vi "testSHA384.vi"(8 "error in (no error)":errorcluster, 11 "TestCase in":refnum<class "TestHashing.lvclass">) -> (0 "error out":errorcluster, 3 "TestCase out":refnum<class "TestHashing.lvclass">)   [LabVIEW 2021, in "TestHashing.lvclass"]
uses:
  TestHashing.lvclass
  TestHashing.lvclass/TestHashing.ctl
  <vilib>/addons/_JKI Toolkits/VI Tester/TestCase.llb/TestCase.lvclass
  <vilib>/Wiresmith Technology/VITAC (VI Tester Advanced Comparisons)/VITAC.lvlib
  C:/Program Files (x86)/National Instruments/LabVIEW 2021/vi.lib/addons/_JKI Toolkits/VI Tester/TestCase.llb/TestCase.lvclass
  Hashing/dotNET Crypto Hashing.lvlib
  Utility/dotNET Crypto Utility.lvlib
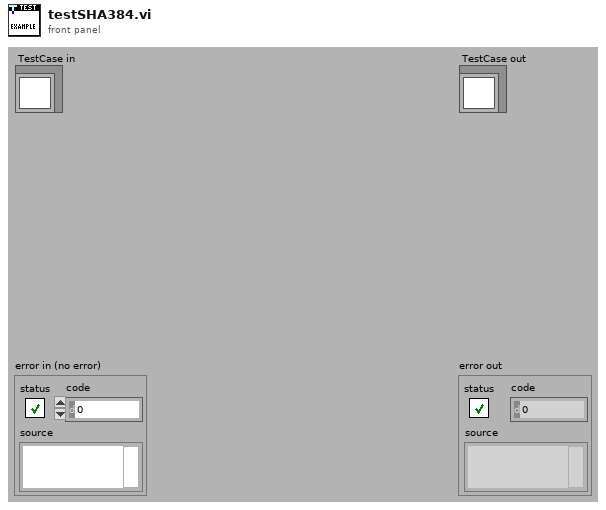
[diagram p1: front panel]
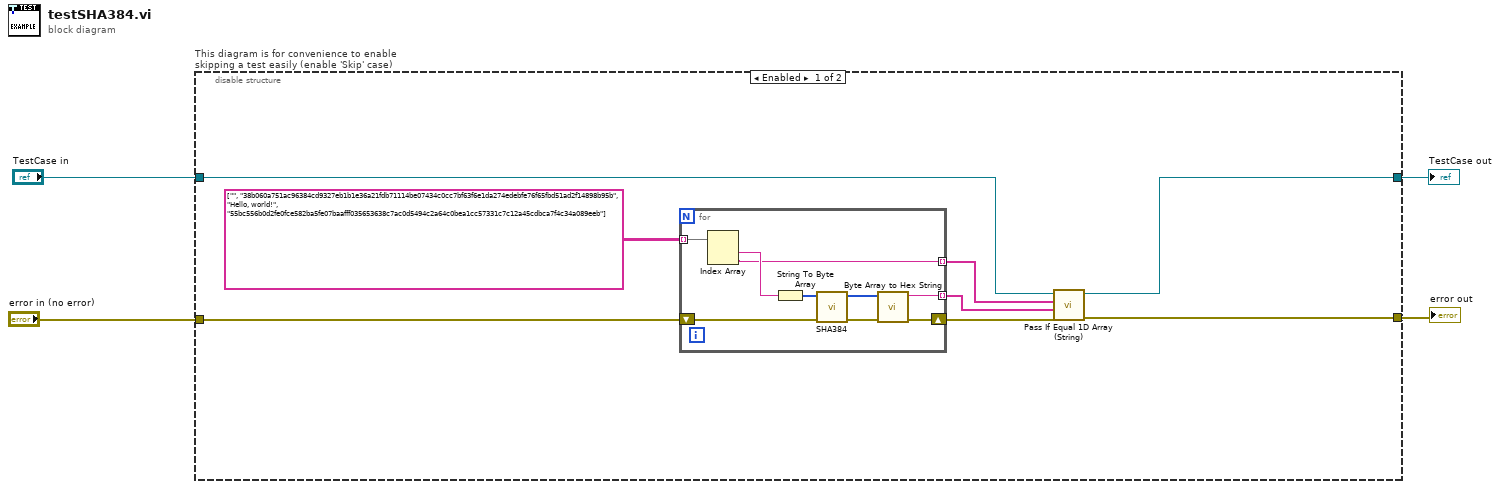
[diagram p0: block diagram]
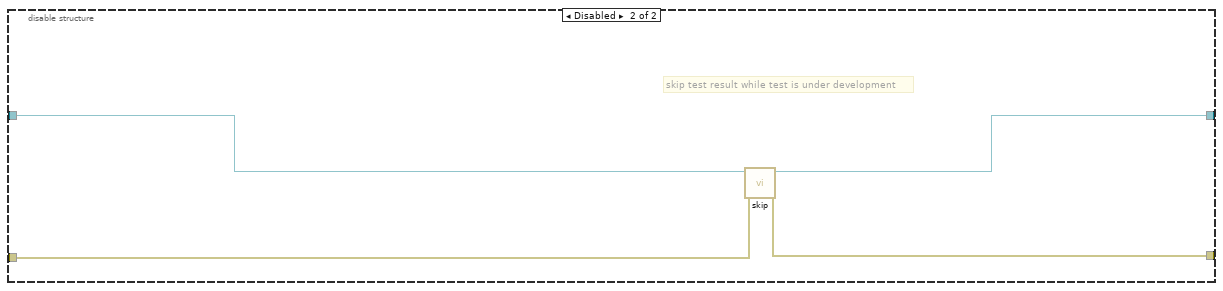
[diagram p2: hidden frame]
diagram:
  n1 = disable-structure "This diagram is for convenience to enable skipping a test easily (enable 'Skip' case)" shown="Enabled" {
    disable-tunnel: "TestCase in" -> [w12 w24]
    disable-tunnel: [w11 w22] -> w1
    disable-tunnel: [w10 w23] -> w3
    disable-tunnel: "error in (no error)" -> [w9 w21]
    frame Enabled {
      n2 = for {
        shift-right: [w19] -> w8
        shift-left: w9 -> [w20]
        tunnel: [w14] -> w7 mode=indexing
        tunnel: string[][] [["", "38b060a751ac96384cd9327eb1b1e36a21fdb71114be07434c0cc7bf63f6e1da274edebfe76f65fbd51ad2f14898b95b"], ["Hello, world!", "55bc556b0d2fe0fce582ba5fe07baafff035653638c7ac0d5494c2a64c0bea1cc57331c7c12a45cdbca7f4c34a089eeb"]] -> [w17] mode=indexing
        tunnel: [w15] -> w5 mode=indexing
        n3 = Index Array(array=w17) -> (element #1=w16:string, element #2=w15:string)  [unwired: 2 in]
        n4 = String To Byte Array(string=w16) -> (unsigned byte array=w13:u8[])
        n5 = call "SHA384.vi"("error in (no error)"=w20, "Data in"=w13) -> ("error out"=w19:errorcluster, "SHA384 Hash"=w18:u8[])  [unwired: 8 in]
        n6 = call "Byte Array to Hex String.vi"("Byte Array"=w18) -> ("Hex String"=w14:string)  [unwired: 10 in]
      }
      n7 = call <vilib>:"Pass If Equal 1D Array (String).vi"("error in (no error)"=w8, "actual"=w7, "expected"=w5, "TestCase in"=w12) -> ("error out"=w10:errorcluster, "TestCase out"=w11:refnum<class "TestHashing.lvclass">)  [unwired: 6 in]
    }
    frame Disabled {
      # "skip test result while test is under development"
      n8 = call <vilib>:"skip.vi"("error in (no error)"=w21, "TestCase in"=w24) -> ("error out"=w23:errorcluster, "TestCase out"=w22:refnum<class "TestHashing.lvclass">)  [unwired: 8 in]
    }
  }
  "error out" <- w3
  "TestCase out" <- w1
